vi "util_multline_comment_hash.vi"(1 "input string":string) -> (0 "result string":string)   [LabVIEW 2020]
doc: "Format a multiline string by prepending a hash character and whitespace padding before the next lines."
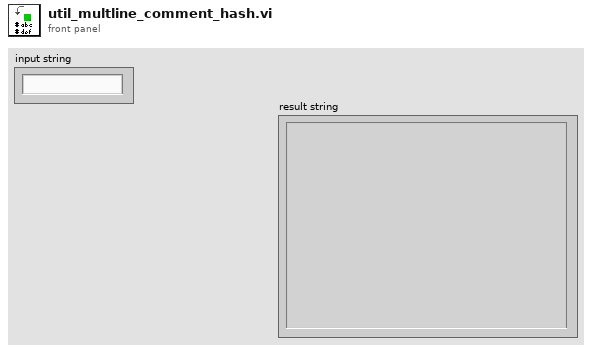
[diagram p1: front panel]
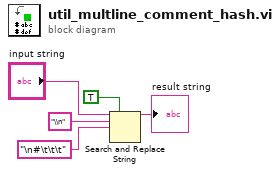
[diagram p0: block diagram]
diagram:
  n1 = Search and Replace String(replace all?=TRUE ("replace all? (F)"), input string="input string", search string="\\n", replace string="\n#\t\t\t" ("replace string (\"\")")) -> (result string=→"result string":string)  [unwired: 4 in, 3 out]
